vi "INITIALIZE.vi"(8 "error in (no error)":errorcluster, 11 "BD_PAPAS_MEX_ESP in":refnum<class "BD_PAPAS_MEX_ESP.lvclass">) -> (0 "error out":errorcluster, 3 "BD_PAPAS_MEX_ESP out":refnum<class "BD_PAPAS_MEX_ESP.lvclass">)   [LabVIEW 2019, in "BD_PAPAS_MEX_ESP.lvlib" / "BD_PAPAS_MEX_ESP.lvclass"]
uses:
  BD_PAPAS_MEX_ESP.lvclass
  BD_PAPAS_MEX_ESP.lvclass/BD_PAPAS_MEX_ESP.ctl
  Read MERCANCIA.vi
  Read VI Refnum.vi
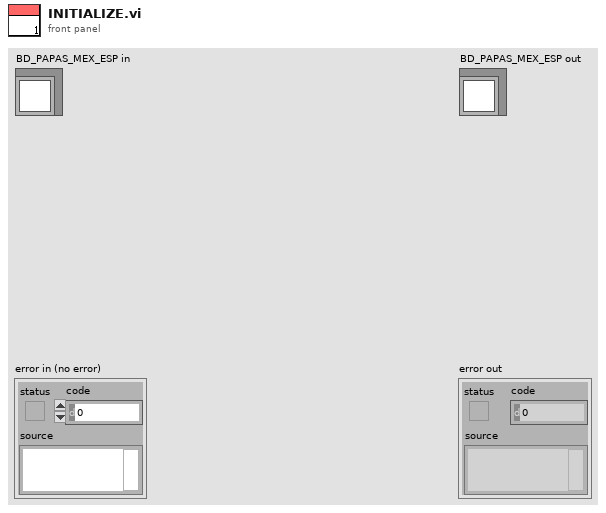
[diagram p1: front panel]
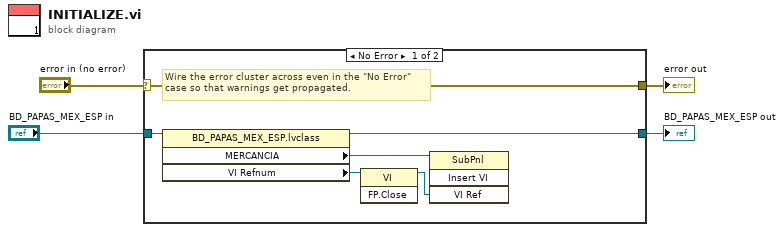
[diagram p0: block diagram]
diagram:
  n1 = case shown="No Error" "error in (no error)" {
    selector: "error in (no error)" -> [w9 w12]
    tunnel: [w9 w12] -> w3
    tunnel: [w8 w11] -> w1
    tunnel: "BD_PAPAS_MEX_ESP in" -> [w10 w11]
    frame No Error {
      # "Wire the error cluster across even in the \"No Error\"\ncase so that warnings get propagated."
      n2 = property class="BD_PAPAS_MEX_ESP.lvclass"(reference=w10) -> (reference out=w8:refnum<class "BD_PAPAS_MEX_ESP.lvclass">, "MERCANCIA"=w6:refnum<vi>, "VI Refnum"=w7:refnum<vi>)  [unwired: 1 in, 1 out]
      n3 = invoke class="VI" method="FP.Close"(reference=w7) -> (reference out=w5:refnum<vi>)  [unwired: 2 in, 2 out]
      n4 = invoke class="SubPnl" method="Insert VI"(reference=w6, "VI Ref"=w5) -> ()  [unwired: 2 in, 4 out]
    }
    frame Error {
    }
  }
  "error out" <- w3
  "BD_PAPAS_MEX_ESP out" <- w1
